vi "6.1.vi"   [LabVIEW 2017]
types:
  T1 = enum16{"open", "replace", "create", "open or create", "replace or create", "replace or create with confirmation"}
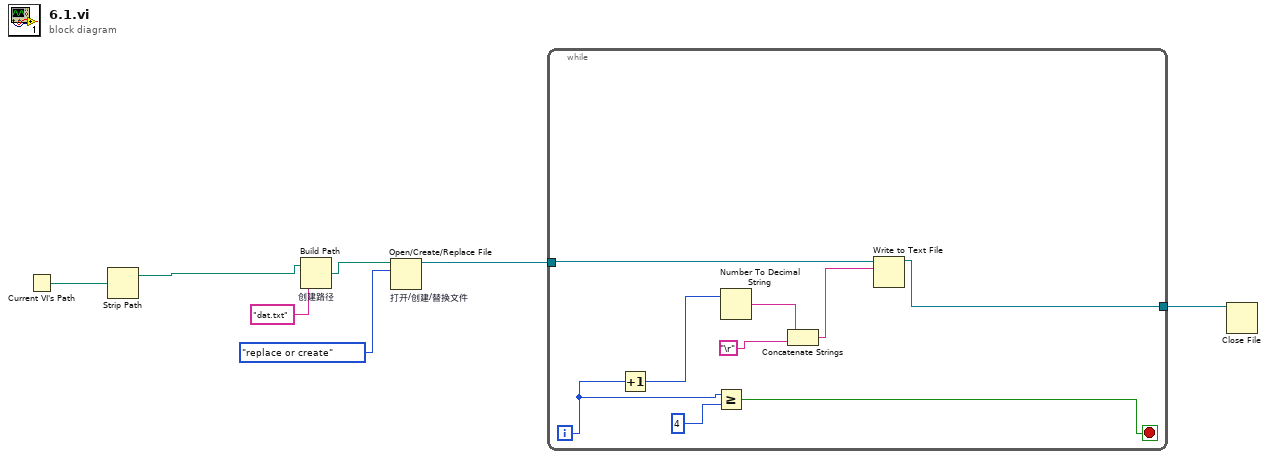
[diagram p0: block diagram]
diagram:
  n1 = Current VI's Path() -> (path=w5:path)
  n2 = Strip Path(path=w5) -> (stripped path=w6:path)  [unwired: 1 out]
  n3 = Build Path "创建路径"(base path=w6, name or relative path="dat.txt" ("名称或相对路径")) -> (appended path=w7:path)
  n4 = Open/Create/Replace File "打开/创建/替换文件"(file path (use dialog)=w7, operation (0:open)=T1."replace or create" ("操作(0:open)")) -> (refnum out=w2:refnum<file>)  [unwired: 4 in, 2 out]
  n5 = while {
    tunnel: w2 -> [w9]
    tunnel: [w8] -> w1
    i -> [w12]
    stop <- w10 stop-if-true
    n6 = Increment(x=w12) -> (x+1=w16:i32)
    n7 = Greater Or Equal?(x=w12, y=4) -> (x >= y?=w10:bool)
    n8 = Number To Decimal String(number=w16) -> (decimal integer string=w15:string)  [unwired: 1 in]
    n9 = Concatenate Strings(w15, "\r") -> (w13:string)
    n10 = Write to Text File(file (use dialog)=w9, text=w13) -> (refnum out=w8:refnum<file>)  [unwired: 2 in, 2 out]
  }
  n11 = Close File(refnum=w1) -> ()  [unwired: 1 in, 2 out]
